vi "FPGA_Wait_Idle.vi"(4 "Times":u32=1000, 5 "Bit_Offset":u32, 6 "Flag":u32, 7 "Offset":u32, 8 "Error_In":errorcluster, 11 "VISA_Rsrc_In":refnum<visa-resource-name>) -> (0 "Error_Out":errorcluster, 3 "VISA_Rsrc_Out":refnum<visa-resource-name>)   [LabVIEW 2018]
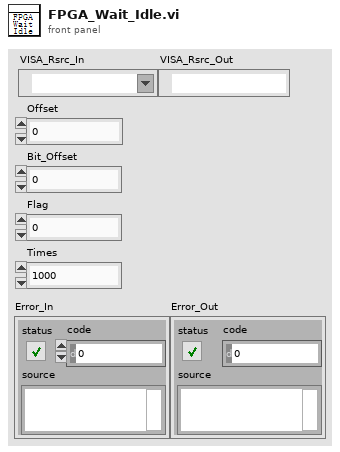
[diagram p1: front panel]
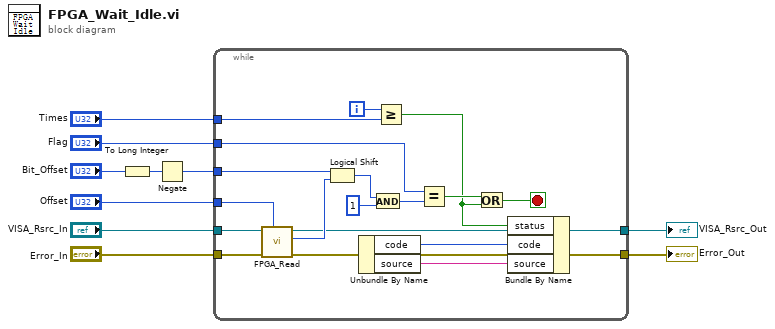
[diagram p0: block diagram]
diagram:
  n1 = To Long Integer(number="Bit_Offset") -> (32bit integer=w7:i32)
  n2 = Negate(x=w7) -> (-x=w5:i32)
  n3 = while {
    tunnel: "VISA_Rsrc_In" -> [w29]
    tunnel: "Error_In" -> [w28]
    tunnel: "Offset" -> [w27]
    tunnel: w5 -> [w26]
    tunnel: "Flag" -> [w21]
    tunnel: [w17] -> w1
    tunnel: "Times" -> [w12]
    tunnel: [w11] -> w2
    i -> [w20]
    stop <- w18 stop-if-true
    n4 = call "FPGA_Read.vi"("Offset"=w27, "Error_In"=w28, "VISA_Rsrc_In"=w29) -> ("Error_Out"=w13:errorcluster, "Value"=w25:u32, "VISA_Rsrc_Out"=w11:refnum<visa-resource-name>)  [unwired: 6 in]
    n5 = Logical Shift(y=w26, x=w25) -> (x << y=w24:u32)
    n6 = Unbundle By Name(w13) -> ("code"=w15:i32, "source"=w14:string)
    n7 = And(x=w24, y=u32 1) -> (x .and. y?=w22:u32)
    n8 = Greater Or Equal?(x=w20, y=w12) -> (x >= y?=w16:bool)
    n9 = Equal?(x=w21, y=w22) -> (x = y?=w19:bool)
    n10 = Or(x=w19, y=w16) -> (x .or. y?=w18:bool)
    n11 = Bundle By Name(cluster=w13, "status"=w16, "code"=w15, "source"=w14) -> (w17:errorcluster)
  }
  "Error_Out" <- w1
  "VISA_Rsrc_Out" <- w2
